vi "Create Board.vi"(9 "ColorBoard":u32(colorbox)=16728794, 10 "BoardSize":cluster{"X":i32, "Y":i32}={"X"=10, "Y"=10}) -> (0 "error out":errorcluster, 3 "Board_Game out":refnum<class "Board_Game.lvclass">)   [LabVIEW 2021, in "Board_Game.lvclass"]
uses:
  Board_Game.lvclass
  Board_Game.lvclass/Board_Game.ctl
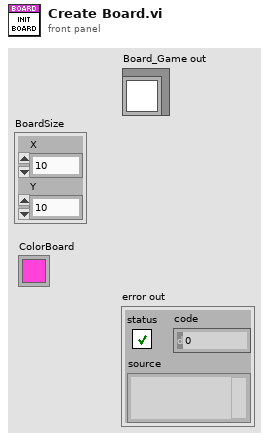
[diagram p1: front panel]
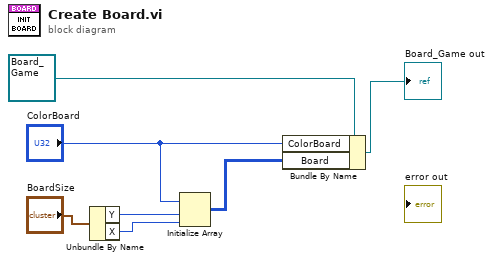
[diagram p0: block diagram]
diagram:
  n1 = Unbundle By Name("BoardSize") -> ("Y"=w1:i32, "X"=w2:i32)
  n2 = Initialize Array("ColorBoard", w1, w2) -> (w4:u32[][])
  n3 = Bundle By Name(cluster=refnum<class "Board_Game.lvclass"> refnum ("Board_Game.lvclass"), "ColorBoard"="ColorBoard", "Board"=w4) -> (→"Board_Game out":refnum<class "Board_Game.lvclass">)
